vi "vettore.vi"(1 "n":u32=6, 2 "fine":dbl=6.0 min=0.0, 3 "inizio":dbl=1.0 min=0.0) -> (0 "Array":dbl[](array[numeric]))   [LabVIEW 2018]
panel:
  in  "ordinato":bool
  out "Waveform Graph":dbl[](graph)
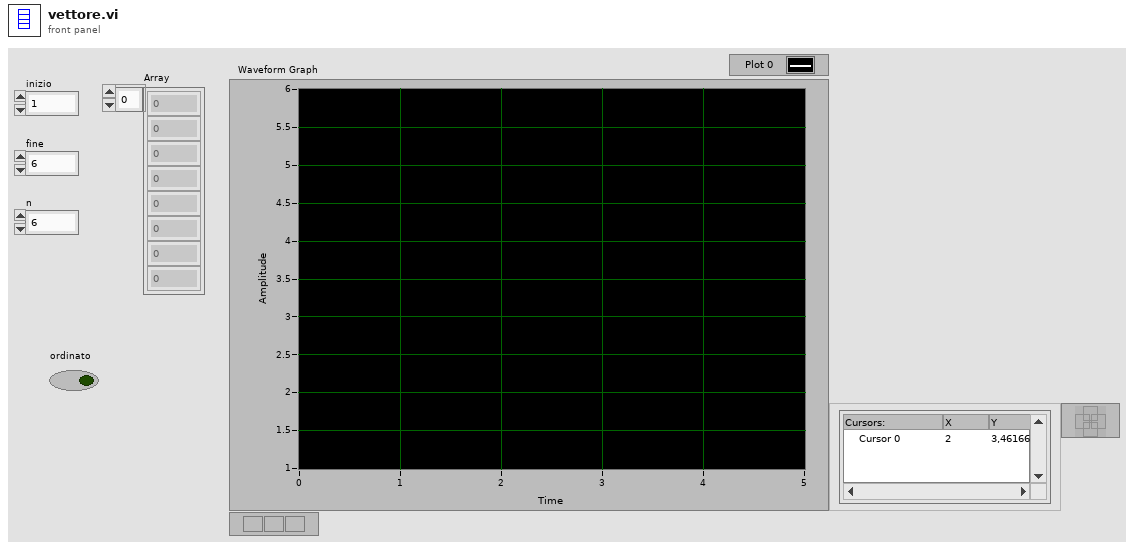
[diagram p1: front panel]
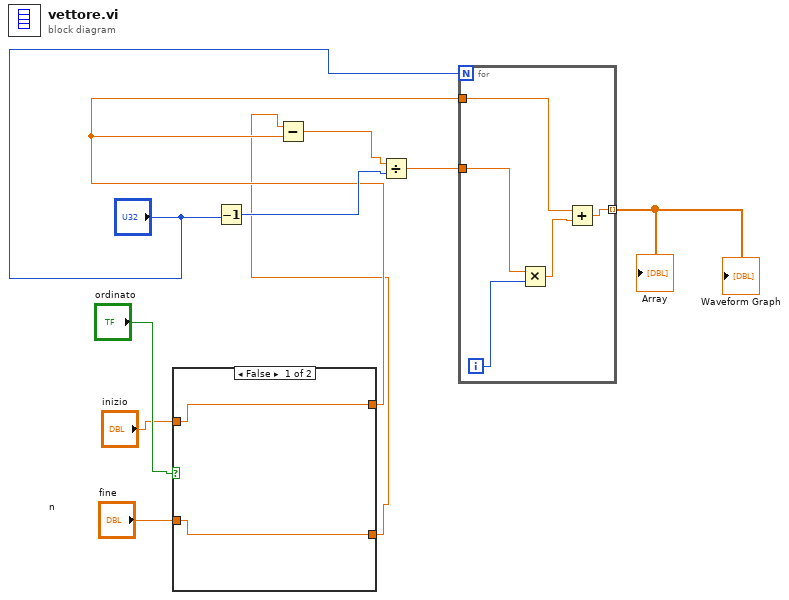
[diagram p0: block diagram]
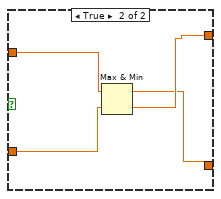
[diagram p2: hidden frame]
diagram:
  n1 = case shown="False" "ordinato" {
    tunnel: "inizio" -> [w12 w16]
    tunnel: "fine" -> [w11 w15]
    tunnel: [w12 w14] -> w2
    tunnel: [w11 w13] -> w1
    frame False {
    }
    frame True {
      n2 = Max & Min(x=w16, y=w15) -> (max(x,y)=w13:dbl, min(x,y)=w14:dbl)
    }
  }
  n3 = Decrement(x="n") -> (x-1=w10:u32)
  n4 = Subtract(x=w1, y=w2) -> (x-y=w9:dbl)
  n5 = Divide(x=w9, y=w10) -> (x/y=w7:dbl)
  n6 = for {
    N: "n" -> [_]
    tunnel: w7 -> [w20]
    tunnel: w2 -> [w18]
    tunnel: [w17] -> w6 mode=indexing
    i -> [w21]
    n7 = Multiply(x=w20, y=w21) -> (x*y=w19:dbl)
    n8 = Add(x=w18, y=w19) -> (x+y=w17:dbl)
  }
  "Array" <- w6
  "Waveform Graph" <- w6
